vi "To JSON.vi"(8 "error in":errorcluster, 11 "RPDO Communication Parameter in":refnum<class "RPDO Communication Parameter.lvclass">) -> (0 "error out":errorcluster, 2 "<JSON>":string, 3 "RPDO Communication Parameter out":refnum<class "RPDO Communication Parameter.lvclass">)   [LabVIEW 2020, in "CANopen.lvlib" / "RPDO Communication Parameter.lvclass"]
uses:
  RPDO Communication Parameter.lvclass
  RPDO Communication Parameter.lvclass/RPDO Communication Parameter.ctl
  340cf549-c0f8-4db1-a607-e4b43f463e50.vi
  <vilib>/JDP Science/JSONtext/Variant to JSON Text.vi
  <vilib>/JDP Science/JSONtext/Set Multiple Object Items.vi
  PDO Communication Parameter/PDO Communication Parameter.lvclass
  <vilib>/JDP Science/JSONtext/LVClass Serializer/JSONtext LVClass Serializer.lvclass
  <vilib>/JDP Science/JSONtext/JSONtext.lvlib
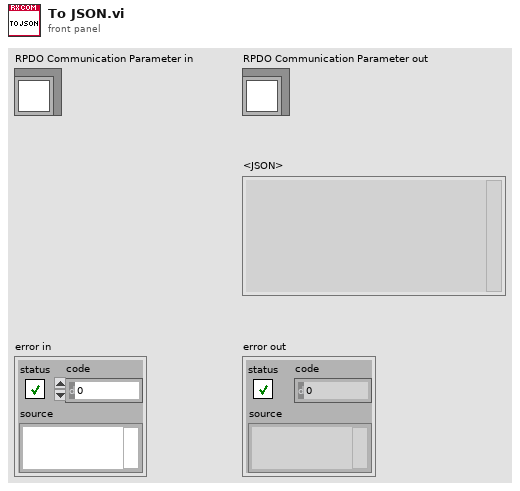
[diagram p1: front panel]
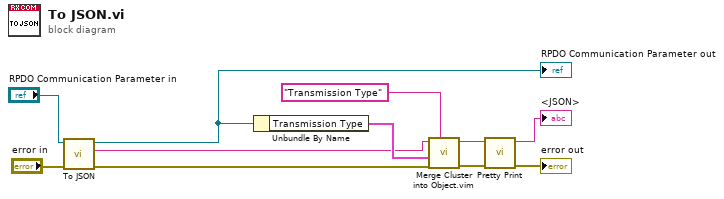
[diagram p0: block diagram]
diagram:
  n1 = call-parent "To JSON.vi"("error in"="error in", "PDO Communication Parameter in"="RPDO Communication Parameter in") -> ("error out"=w8:errorcluster, "<JSON>"=w4:string, "PDO Communication Parameter out"=w9:refnum<class "RPDO Communication Parameter.lvclass">)  [unwired: 7 in]
  "RPDO Communication Parameter out" <- w9
  n2 = Unbundle By Name(w9) -> ("Transmission Type"=w6:cluster{"Null":bool, "Value":u8})
  n3 = call "Merge Cluster into Object.vim"("$Path or Item Name"="Transmission Type", "error in (no error)"=w8, "Any Cluster"=w6, "JSON"=w4) -> ("error out"=w7:errorcluster, "<JSON>"=w2:string)  [unwired: 5 in]
  n4 = call <vilib>:"Pretty Print.vi"("error in (no error)"=w7, "JSON"=w2) -> ("error out"=→"error out":errorcluster, "<JSON>"=→"<JSON>":string)  [unwired: 7 in, 1 out]
